vi "Find MHL Frames.vi"(8 "error in":errorcluster, 10 "Event Name":string, 11 "References":refnum<vi>[](array[refnum])) -> (0 "error out":errorcluster)   [LabVIEW 2019, in "Panther Dashboard.lvlib"]
uses:
  Panther Dashboard.lvlib
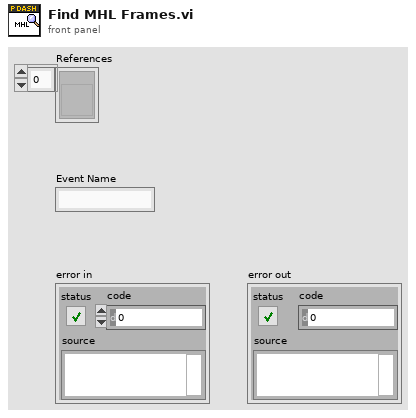
[diagram p1: front panel]
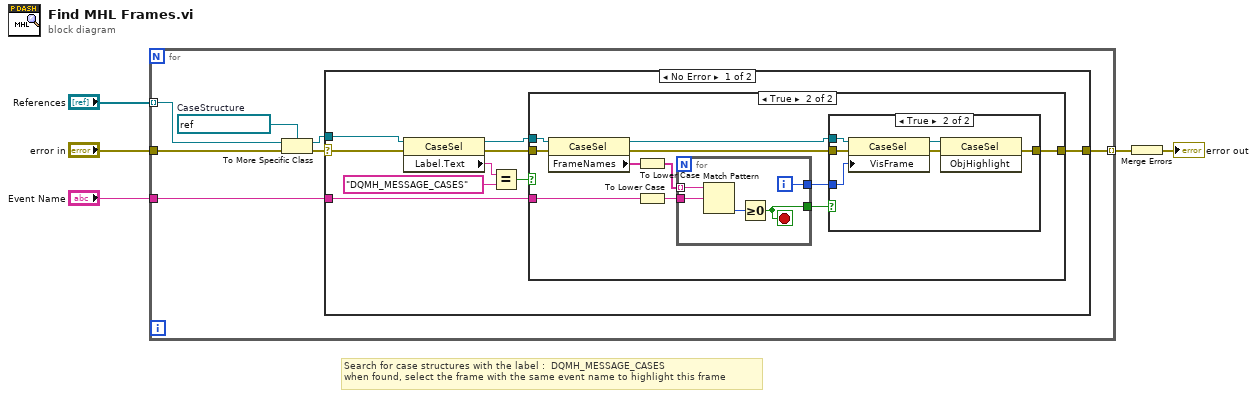
[diagram p0: block diagram]
diagram:
  # "Search for case structures with the label :  DQMH_MESSAGE_CASES\nwhen found, select the frame with the same event name to highlight this frame"
  n1 = for {
    tunnel: "References" -> [w9] mode=indexing
    tunnel: [w11] -> w1 mode=indexing
    tunnel: "Event Name" -> [w6]
    tunnel: "error in" -> [w10]
    w8 = refnum<vi> refnum  # CaseStructure
    n2 = To More Specific Class(target class=w8, reference=w9, error in=w10) -> (specific class reference=w7:refnum<vi>, error out=w12:errorcluster)
    n3 = case shown="No Error" w12 {
      selector: w12 -> [w20 _]
      tunnel: w7 -> [w18 _]
      tunnel: [w21 _] -> w11
      tunnel: w6 -> [w14 _]
      frame No Error {
        n4 = property class="CaseSel"(reference=w18, error in=w20) -> (reference out=w15:refnum<vi>, error out=w19:errorcluster, "Label.Text"=w13:string)
        n5 = Equal?(x=w13, y="DQMH_MESSAGE_CASES") -> (x = y?=w16:bool)
        n6 = case shown="True" w16 {
          tunnel: [w22 w33] -> w21
          tunnel: w15 -> [_ w30]
          tunnel: w14 -> [_ w25]
          tunnel: w19 -> [w22 w32]
          frame False {
          }
          frame True {
            n7 = property class="CaseSel"(reference=w30, error in=w32) -> (reference out=w27:refnum<vi>, error out=w31:errorcluster, "FrameNames"=w29:string[])
            n8 = To Lower Case(string=w29) -> (all lower case string=w23:string[])
            n9 = To Lower Case(string=w25) -> (all lower case string=w24:string)
            n10 = for {
              tunnel: w23 -> [w41] mode=indexing
              tunnel: w24 -> [w44]
              tunnel: [w45] -> w28
              tunnel: [w42] -> w26
              i -> [w45]
              stop <- w42 stop-if-true
              n11 = Match Pattern(string=w41, regular expression=w44) -> (offset past match=w43:i32)  [unwired: 1 in, 3 out]
              n12 = Greater Or Equal To 0?(x=w43) -> (x >= 0?=w42:bool)
            }
            n13 = case shown="True" w26 {
              tunnel: [w34 w39] -> w33
              tunnel: w31 -> [w34 w38]
              tunnel: w28 -> [_ w36]
              tunnel: w27 -> [_ w35]
              frame False {
              }
              frame True {
                n14 = property class="CaseSel"(reference=w35, error in=w38, "VisFrame"=w36) -> (reference out=w37:refnum<vi>, error out=w40:errorcluster)
                n15 = invoke class="CaseSel" method="ObjHighlight"(reference=w37, error in=w40) -> (error out=w39:errorcluster)  [unwired: 1 in, 2 out]
              }
            }
          }
        }
      }
      frame Error {
      }
    }
  }
  n16 = Merge Errors(w1) -> (→"error out":errorcluster)
